vi "Send Event Generated.vi"(5 "Message Type":refnum<class "Event Generated Msg.lvclass">, 7 "Message Priority (Normal)":T1=enum."Normal", 8 "Error In":errorcluster, 10 "Event Data":refnum<class "Event.lvclass">, 11 "Message Enqueuer":refnum<class "Message Enqueuer.lvclass">) -> (0 "Error Out":errorcluster, 3 "Message Enqueuer Out":refnum<class "Message Enqueuer.lvclass">)   [LabVIEW 2019, in "Event Source.lvlib" / "Event Generated Msg.lvclass"]
doc: "This is a method used to publish the event data to all registered actors. It can be only called inside the Event Source Actor."
uses:
  Event Generated Msg.lvclass
  <vilib>/ActorFramework/Message Enqueuer/Message Enqueuer.lvclass
  <vilib>/ActorFramework/Message Enqueuer/Message Priority.ctl
  C:/Program Files/National Instruments/LabVIEW 2019/vi.lib/ActorFramework/Message/Message.lvclass
  Event/Event.lvclass
  Event Generated Msg.lvclass/Event Generated Msg.ctl
  <vilib>/ActorFramework/Message Enqueuer/Message Enqueuer.lvclass/Message Enqueuer.ctl
  <vilib>/ActorFramework/Message Priority Queue/Priority Enqueue.vi
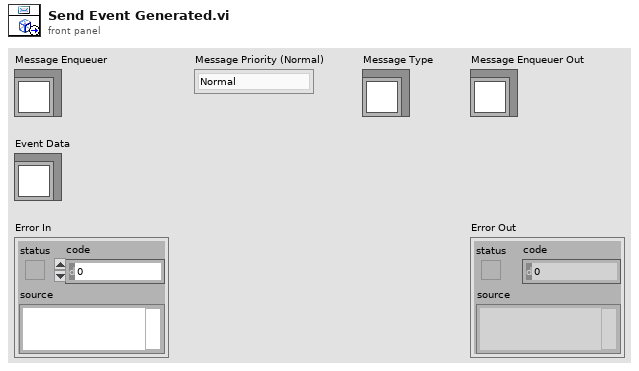
[diagram p1: front panel]
types:
  T1 = typedef "Actor Framework.lvlib/Message Enqueuer.lvclass/Message Priority.ctl" = enum16{"Low", "Normal", "High"}
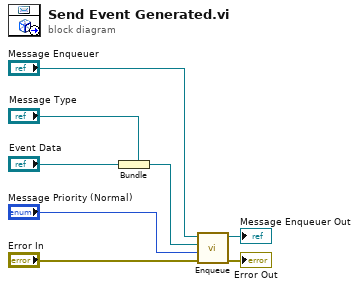
[diagram p0: block diagram]
diagram:
  n1 = Bundle(cluster="Message Type", "Event Data") -> (w4:refnum<class "Event Generated Msg.lvclass">)
  n2 = call <vilib>:"Enqueue.vi"("error in (no error)"="Error In", "Message Priority (Normal)"="Message Priority (Normal)", "Message"=w4, "Message Enqueuer in"="Message Enqueuer") -> ("error out"=→"Error Out":errorcluster, "Message Enqueuer out"=→"Message Enqueuer Out":refnum<class "Message Enqueuer.lvclass">)  [unwired: 6 in]
